vi "Subtract.vi"(1 "Vec2 b in":refnum<class "Vector2.lvclass">, 2 "Vec2 a in":refnum<class "Vector2.lvclass">) -> (0 "Vec2 out":refnum<class "Vector2.lvclass">)   [LabVIEW 2022 SP3, in "Vector2.lvclass"]
uses:
  Vector2.lvclass
  Vector2.lvclass/Vector2.ctl
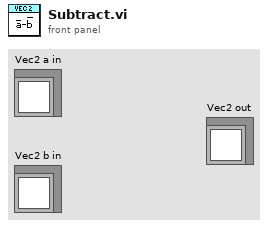
[diagram p1: front panel]
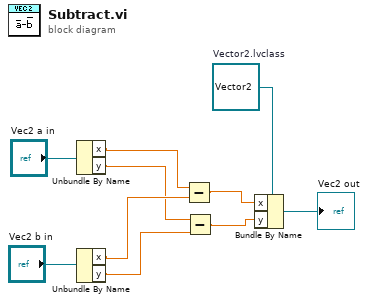
[diagram p0: block diagram]
diagram:
  w4 = refnum<class "Vector2.lvclass"> refnum  # Vector2.lvclass
  n1 = Unbundle By Name("Vec2 a in") -> ("x"=w8:dbl, "y"=w6:dbl)
  n2 = Unbundle By Name("Vec2 b in") -> ("x"=w7:dbl, "y"=w5:dbl)
  n3 = Subtract(x=w8, y=w7) -> (x-y=w3:dbl)
  n4 = Subtract(x=w6, y=w5) -> (x-y=w2:dbl)
  n5 = Bundle By Name(cluster=w4, "x"=w3, "y"=w2) -> (→"Vec2 out":refnum<class "Vector2.lvclass">)
